vi "Profile Main to Loop.vi"(0 "Run Profile":bool, 1 "Test Profile (FPGA)":T1[](array[typedef]), 2 "Profile Steps":u8, 3 "Current Step":u8, 4 "Step Time Left":u32, 5 "Error IN":errorcluster, 8 "Write (F)":bool) -> (14 "Run Profile OUT":bool, 15 "Test Profile (FPGA) OUT":T1[](array[typedef]), 16 "Profile Steps OUT":u8, 17 "Current Step OUT":u8, 18 "Step Time Left OUT":u32, 19 "Error OUT":errorcluster)   [LabVIEW 2019]
uses:
  Type Defs/Test Step (FPGA).ctl
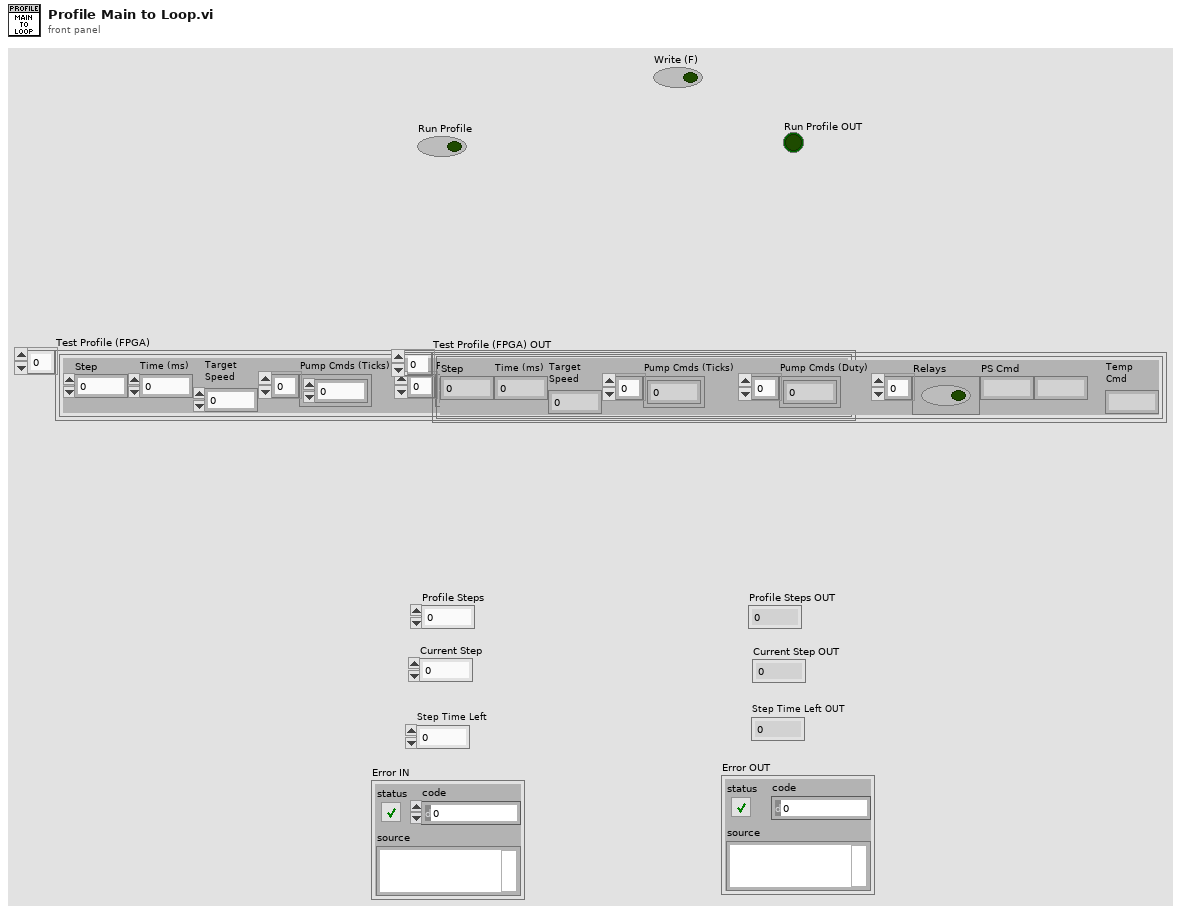
[diagram p1: front panel]
types:
  T1 = typedef "Test Step (FPGA).ctl" = cluster{"Step":u8, "Time (ms)":u32, "Target\nSpeed":u16, "Pump Cmds (Ticks)":i32[], "Pump Cmds (Duty)":u32[], "Relays":bool[], "PS Cmd":fxp<+/-,20,5>, "Pressure Cmd":fxp<+/-,20,5>, "Temp\nCmd":i16}
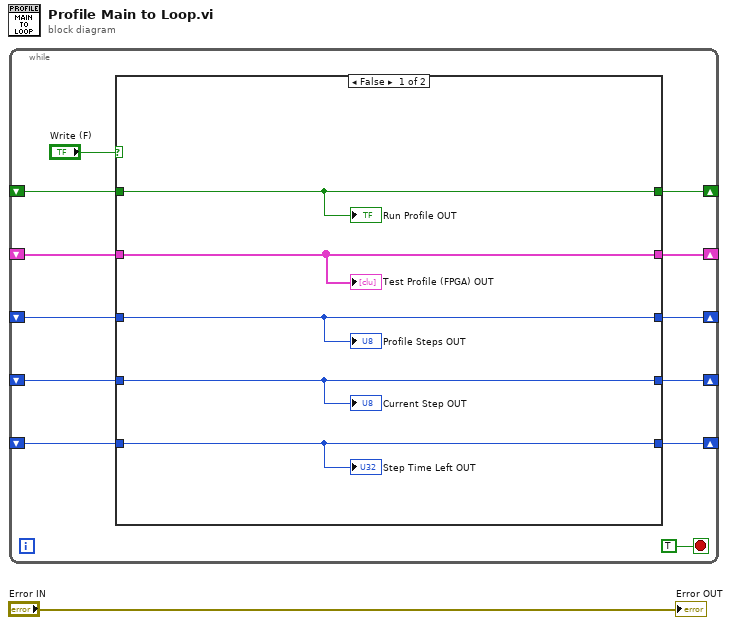
[diagram p0: block diagram]
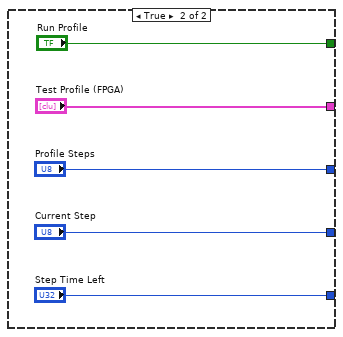
[diagram p2: hidden frame]
diagram:
  n1 = while {
    shift-right: [w11] -> _
    shift-left: _ -> [w6]
    shift-right: [w10] -> _
    shift-left: _ -> [w5]
    shift-right: [w9] -> _
    shift-left: _ -> [w4]
    shift-right: [w8] -> _
    shift-left: _ -> [w3]
    shift-right: [w7] -> _
    shift-left: _ -> [w2]
    stop <- TRUE stop-if-true
    n2 = case shown="False" "Write (F)" {
      tunnel: [w18 "Run Profile"] -> w11
      tunnel: [w17 "Test Profile (FPGA)"] -> w10
      tunnel: [w16 "Profile Steps"] -> w9
      tunnel: [w15 "Current Step"] -> w8
      tunnel: [w14 "Step Time Left"] -> w7
      tunnel: w6 -> [w18 _]
      tunnel: w5 -> [w17 _]
      tunnel: w4 -> [w16 _]
      tunnel: w3 -> [w15 _]
      tunnel: w2 -> [w14 _]
      frame False {
        "Run Profile OUT" <- w18
        "Test Profile (FPGA) OUT" <- w17
        "Profile Steps OUT" <- w16
        "Current Step OUT" <- w15
        "Step Time Left OUT" <- w14
      }
      frame True {
      }
    }
  }
  "Error OUT" <- "Error IN"
